vi "Post-Init.vi"(8 "error in (no error)":errorcluster, 11 "NI-Scope Lock-in Driver in":refnum<class "NI-Scope Lock-in Driver.lvclass">) -> (0 "error out":errorcluster, 2 "Init Result":refnum<class "Acquired Result.lvclass">, 3 "NI-Scope Lock-in Driver out":refnum<class "NI-Scope Lock-in Driver.lvclass">)   [LabVIEW 2019, in "NI-Scope Lock-in Driver.lvclass"]
uses:
  NI-Scope Lock-in Driver.lvclass
  C:/GitHub/NHMFL_Core/Libraries/Instruments/Instrument Driver/Instrument Driver.lvclass
  Instruments/Results/Acquired Result/Acquired Result.lvclass
  Instruments/Instrument Driver/Instrument Driver.lvclass/Instrument Driver.ctl
  Instruments/Results/Acquired Result/Acquired Result.lvclass/Acquired Result.ctl
  Instruments/Instrument Driver/Write Channel units.vi
  Instruments/Instrument Driver/Write Channel names.vi
  Instruments/Results/Acquired Result/Write Channels.vi
  NI-Scope Digitizer/Ni-Scope Digitizer.lvclass
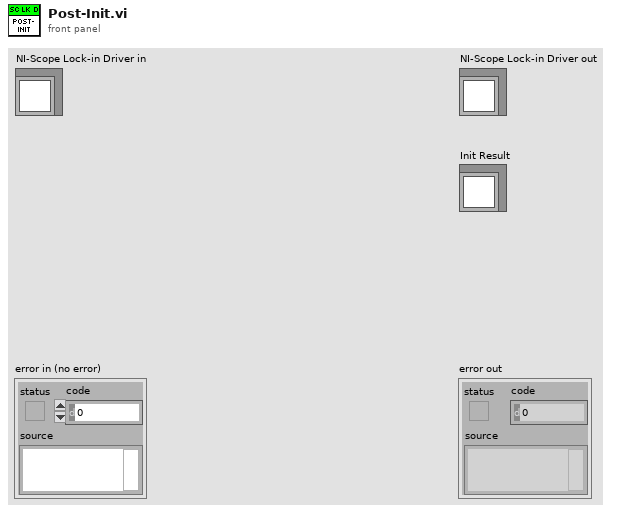
[diagram p1: front panel]
types:
  T1 = typedef "NI-Scope Lock-in Configuration.ctl" = cluster{"Points per sine wave":i32, "Rate":dbl, "Re-name channels":string[], "Active channels":string, "Ranges":dbl[], "Sync on trigger":bool, "R-Q":bool}
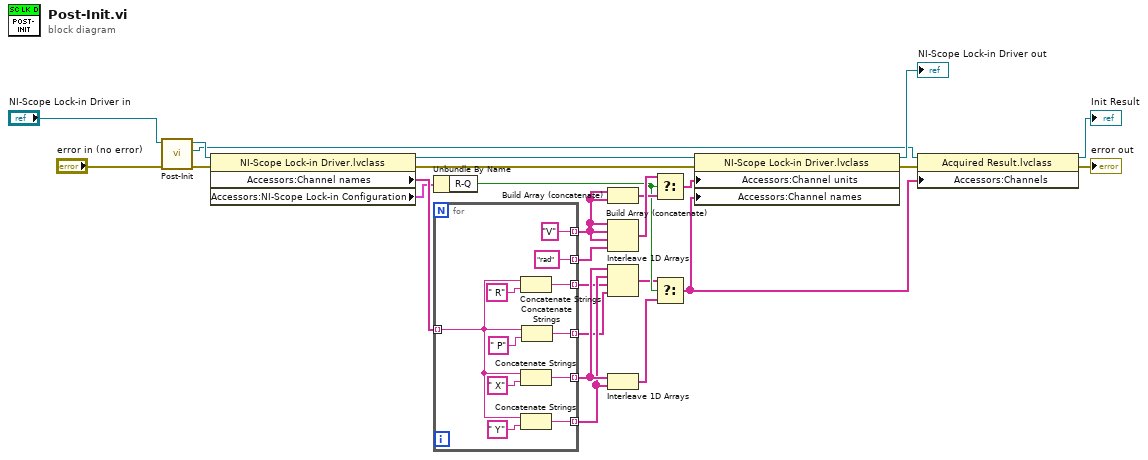
[diagram p0: block diagram]
diagram:
  n1 = call-parent "Post-Init.vi"("error in (no error)"="error in (no error)", "Pulse Driver in"="NI-Scope Lock-in Driver in") -> ("error out"=w26:errorcluster, "Init Result"=w18:refnum<class "Acquired Result.lvclass">, "Pulse Driver out"=w22:refnum<class "NI-Scope Lock-in Driver.lvclass">)  [unwired: 7 in]
  n2 = property class="NI-Scope Lock-in Driver.lvclass"(reference=w22, error in=w26) -> (reference out=w21:refnum<class "NI-Scope Lock-in Driver.lvclass">, error out=w23:errorcluster, "Accessors:Channel names"=w19:string[], "Accessors:NI-Scope Lock-in Configuration"=w12:T1)
  n3 = Unbundle By Name(w12) -> ("R-Q"=w8:bool)
  n4 = for {
    tunnel: w19 -> [w32] mode=indexing
    tunnel: [w35] -> w6 mode=indexing
    tunnel: [w34] -> w5 mode=indexing
    tunnel: ["V" ("string")] -> w13 mode=indexing
    tunnel: [w31] -> w4 mode=indexing
    tunnel: [w30] -> w3 mode=indexing
    tunnel: ["rad" ("string")] -> w14 mode=indexing
    n5 = Concatenate Strings(w32, " R" ("string")) -> (w31:string)
    n6 = Concatenate Strings(w32, " X" ("string")) -> (w35:string)
    n7 = Concatenate Strings(w32, " Y" ("string")) -> (w34:string)
    n8 = Concatenate Strings(w32, " P" ("string")) -> (w30:string)
  }
  n9 = Build Array (concatenate)(w13, w13) -> (w10:string[])
  n10 = Build Array (concatenate)(w13, w13, w13, w14) -> (w11:string[])
  n11 = Interleave 1D Arrays(w6, w5, w4, w3) -> (w2:string[])
  n12 = Interleave 1D Arrays(w6, w5) -> (w7:string[])
  n13 = Select(t=w11, s=w8, f=w10) -> (s? t:f=w9:string[])
  n14 = Select(t=w2, s=w8, f=w7) -> (s? t:f=w1:string[])
  n15 = property class="NI-Scope Lock-in Driver.lvclass"(reference=w21, error in=w23, "Accessors:Channel units"=w9, "Accessors:Channel names"=w1) -> (reference out=→"NI-Scope Lock-in Driver out":refnum<class "NI-Scope Lock-in Driver.lvclass">, error out=w16:errorcluster)
  n16 = property class="Acquired Result.lvclass"(reference=w18, error in=w16, "Accessors:Channels"=w1) -> (reference out=→"Init Result":refnum<class "Acquired Result.lvclass">, error out=→"error out":errorcluster)
